vi "imp_v12p4_theta23_v2.vi"() -> ()   [LabVIEW 2014]
uses:
  <vilib>/FPGAPlugInAG/cRIO-9039/niLvFpga_Open_cRIO-9039.vi
  <vilib>/rvi/interface/common/dynamic/niFpgaDynamicAddResources.vi
  <vilib>/Utility/error.llb/Error Cluster From Error Code.vi
  <vilib>/rvi/errors/niLvFpgaAdjustHostInterfaceError.vi
  <vilib>/imath/engines/lvmath2/RunTimeEngine/BuiltInFunctions/asin/NIMS_asin(C).vi
  <instcachedir>/0/NIMS_asin(C)_7FBCC14D953545E18098594EA458D330.lvgen/NIMS_asin(C)_7FBCC14D953545E18098594EA458D330_001.vi
  <vilib>/imath/engines/lvmath2/RunTimeEngine/BuiltInFunctions/atan2/NIMS_atan2.vi
  <instcachedir>/0/NIMS_atan2_A91AA4A7D42247EDBE8F76DB99AF04A4.lvgen/NIMS_atan2_A91AA4A7D42247EDBE8F76DB99AF04A4_000.vi
  <vilib>/imath/engines/lvmath2/RunTimeEngine/NodeEndStatement/NIMS_NodeEndStatement_Output.vi
  <instcachedir>/0/NIMS_NodeEndStatement_Output_53EC0D466D134D7ABD903AC30B43404B.lvgen/NIMS_NodeEndStatement_Output_53EC0D466D134D7ABD903AC30B43404B_001.vi
  <instcachedir>/0/NIMS_NodeEndStatement_Output_53EC0D466D134D7ABD903AC30B43404B.lvgen/NIMS_NodeEndStatement_Output_53EC0D466D134D7ABD903AC30B43404B_010.vi
  <vilib>/imath/engines/lvmath2/RunTimeEngine/ErrorHandling/NIMS_Finalize Error.vi
  <vilib>/rvi/interface/nirviOpenFPGA/nirviOpenFPGA.xnode
  FPGA Bitfiles/test0304_FPGATarget_imptestv12p4_nHMFqqsr4pc.lvbitx
  FPGA VIs/imp_test_v12_p4.vi
  <vilib>/rvi/interface/nirviReadWriteControl/nirviReadWriteControl.xnode
  <vilib>/rvi/interface/Simulation/niFpgaSimulationCallBeginRW.vi
  NiFpgaLv.dll
panel:
  out "kv2Kv":dbl
  out "theta3_deg":dbl
  out "theta2_deg":cdb
  out "Kv_p":cdb
  out "theta3 (rad)":dbl
  out "theta2 (rad)":dbl
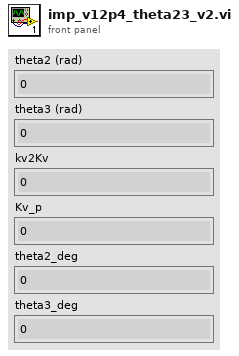
[diagram p1: front panel]
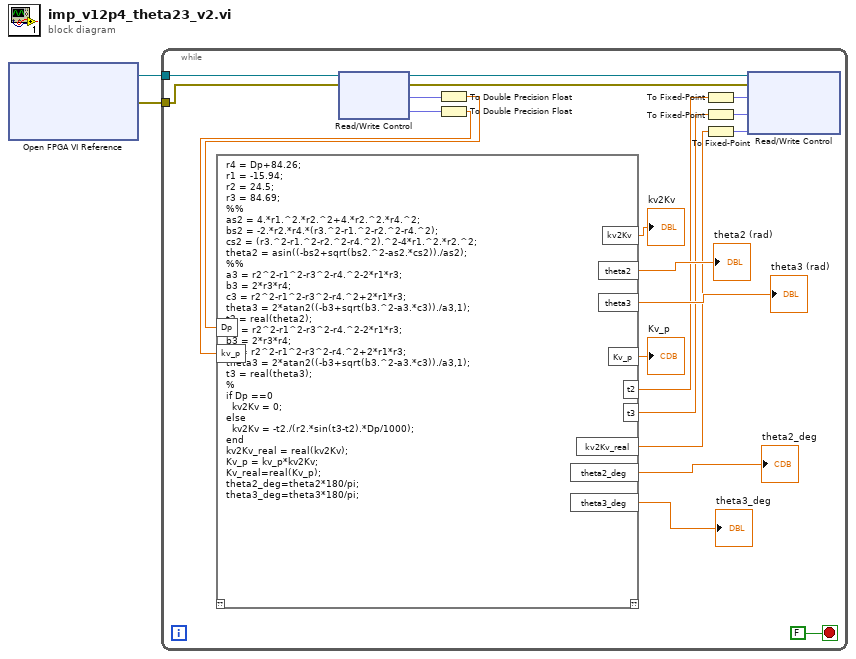
[diagram p0: block diagram]
diagram:
  n1 = xnode "Open FPGA VI Reference"() -> ("FPGA VI Reference Out"=w2:refnum<k20>, "error out"=w1:errorcluster)  [unwired: 2 in]
  n2 = while {
    tunnel: w2 -> [w14]
    tunnel: w1 -> [w21]
    stop <- FALSE stop-if-true
    n3 = xnode "Read/Write Control"("FPGA VI Reference In"=w14, "error in"=w21) -> ("FPGA VI Reference Out"=w13:refnum<k20>, "error out"=w12:errorcluster, "D_p(mm)"=w23:fxp<+/-,32,7>, "kv_p"=w19:fxp<+/-,35,13>)
    n4 = To Double Precision Float(number=w23) -> (double precision float=w22:dbl)
    n5 = To Double Precision Float(number=w19) -> (double precision float=w18:dbl)
    n6 = mathscript code="r4 = Dp+84.26;\nr1 = -15.94;\nr2 = 24.5;\nr3 = 84.69;\n%%\nas2 = 4.*r1.^2.*r2.^2+4.*r2.^2.*r4.^2;\nbs2 = -2.*r2.*r4.*(r3.^2-r1.^2-r2.^2-r4.^2);\ncs2 = (r3.^2-r1.^2-r2.^2-r4.^2).^2-4*r1.^2.*r2.^2;\ntheta2 = asin((-bs2+sqrt(bs2.^2-as2.*cs2))./as2);\n%%\na3 = r2^2-r1^2-r3^2-r4.^2-2*r1*r3;\nb3 = 2*r3*r4;\nc3 = r2^2-r1^2-r3^2-r4.^2+2*r1*r3;\ntheta3 = 2*atan2((-b3+sqrt(b3.^2-a3.*c3))./a3,1);\nt2 = real(theta2);\na3 = r2^2-r1^2-r3^2-r4.^2-2*r1*r3;\nb3 = 2*r3*r4;\nc3 = r2^2-r1^2-r3^2-r4.^2+2*r1*r3;\ntheta3 = 2*atan2((-b3+sqrt(b3.^2-a3.*c3))./a3,1);\nt3 = real(theta3);\n%\nif Dp ==0\n  kv2Kv = 0;\nelse\n  kv2Kv = -t2./(r2.*sin(t3-t2).*Dp/1000);\nend\nkv2Kv_real = real(kv2Kv);\nKv_p = kv_p*kv2Kv;\nKv_real=real(Kv_p);\ntheta2_deg=theta2*180/pi;\ntheta3_deg=theta3*180/pi;"("Dp"=w22, "kv_p"=w18) -> ("theta2"=→"theta2 (rad)":cdb, "theta3"=→"theta3 (rad)":dbl, "Kv_p"=→"Kv_p":dbl, "t2"=w9:dbl, "theta2_deg"=→"theta2_deg":cdb, "theta3_deg"=→"theta3_deg":dbl, "t3"=w6:dbl, "kv2Kv_real"=w5:dbl, "kv2Kv"=→"kv2Kv":dbl)  [unwired: 1 in, 1 out]
    n7 = To Fixed-Point(number=w9) -> (fixed-point=w16:fxp<+/-,32,16>)  [unwired: 1 in]
    n8 = To Fixed-Point(number=w6) -> (fixed-point=w20:fxp<+/-,32,16>)  [unwired: 1 in]
    n9 = To Fixed-Point(number=w5) -> (fixed-point=w17:fxp<+/-,32,16>)  [unwired: 1 in]
    n10 = xnode "Read/Write Control"("FPGA VI Reference In"=w13, "error in"=w12, "theta2p (rad)"=w16, "theta3p (rad)"=w20, "kv2Kv"=w17) -> ()  [unwired: 2 out]
  }
